vi "load_xml.vi"(8 "error in":errorcluster, 10 "child node in":refnum<k20>, 11 "Analog_Output.lvclass (in)":refnum<class "Analog_Output.lvclass">) -> (0 "error out":errorcluster, 2 "child node out":refnum<k20>, 3 "Analog_Output.lvclass":refnum<class "Analog_Output.lvclass">)   [LabVIEW 2014, in "Analog_Output.lvclass"]
doc: "Loads analog output settings from xml. Expected format:\n\n<Enable>%b</Enable>\n<PhysicalChannel>%s</PhysicalChannel>\n<MinimumValue>%f</MinimumValue>\n<MaximumValue>%f</MaximumValue>\n<SamplesPerSecond>%f</SamplesPerSecond>\n<TotalAOTime units=\"seconds\">%s</TotalAOTime>\n<AnalogOutputEquations>\n%s</AnalogOutputEquations>\n<StartTrigger.WaitForStartTrigger>%b</StartTrigger.WaitForStartTrigger\n<StartTrigger.source>%s</StartTrigger.source>\n<StartTrigger.edge>%s</StartTrigger.edge>\n\nMTL 2012 Dec 31"
uses:
  Analog_Output.lvclass
  Analog_Output.lvclass/Analog_Output.ctl
  Globals.vi
  <vilib>/xml/Close Reference(Node).vi
  <resource>/objmgr/DOMUserDefRef.rc
  <vilib>/xml/NI_XML.lvlib
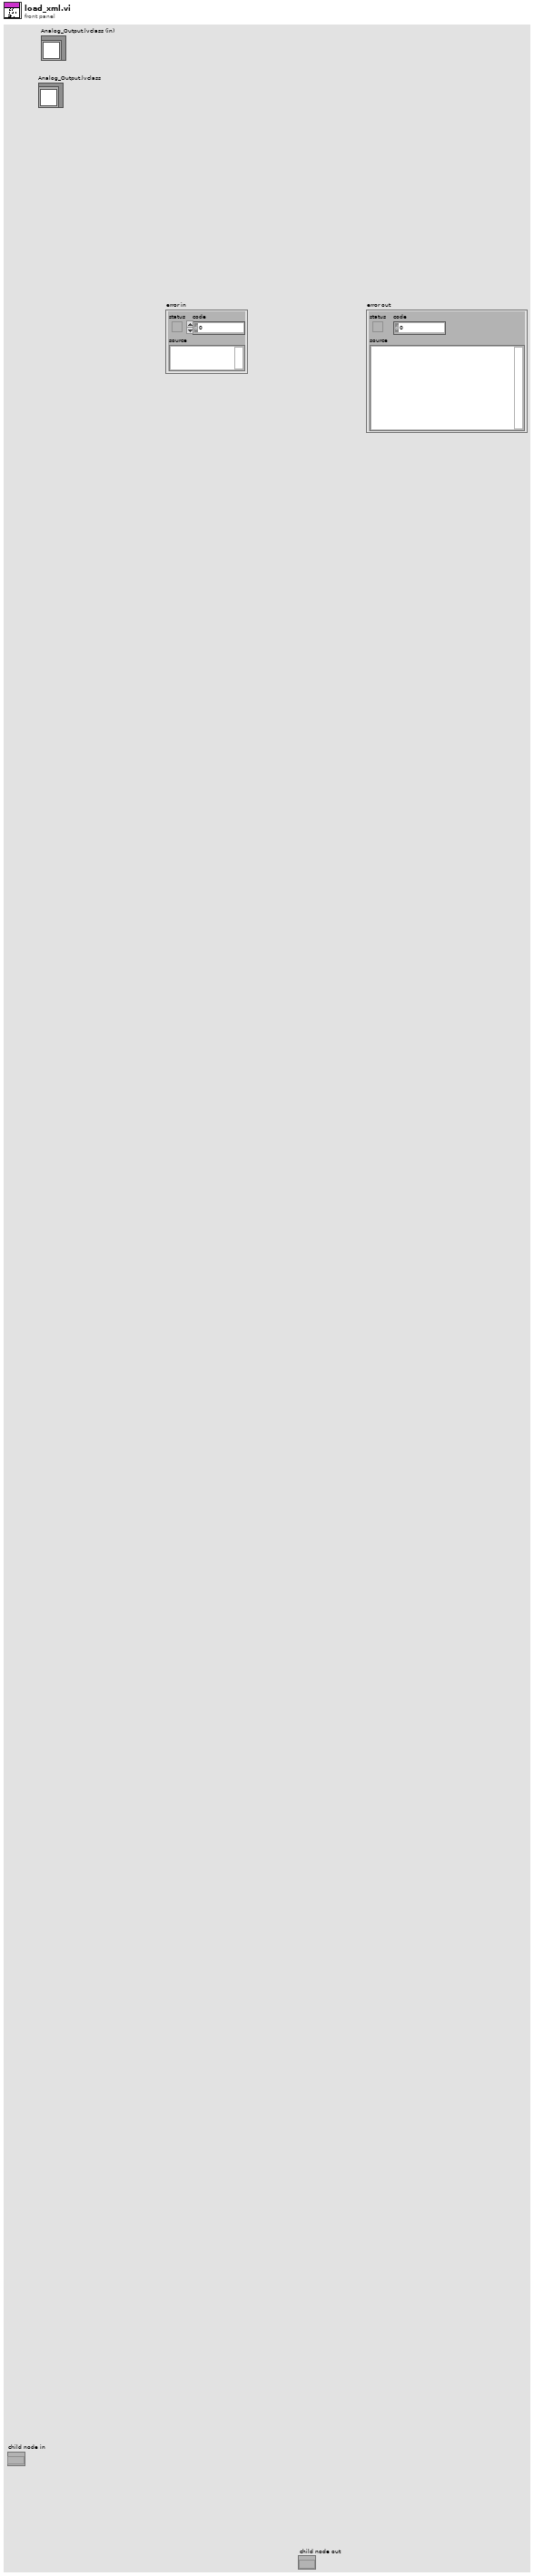
[diagram p1: front panel]
types:
  T1 = typedef "Analog_Output.lvclass/AO_settings.ctl" = cluster{"Enable Analog Out?":bool, "Physical Channel":tag, "Minimum Value":dbl, "Maximum Value":dbl, "Samples per second":dbl, "Start Trigger":cluster{"Wait for start trigger?":bool, "source":tag, "edge":i32}, "Analog Output Waveforms (channel, time)":dbl[][], "Export trigger":cluster{"Export Start Trigger?":bool, "output terminal":tag}, "External Clock":cluster{"Use external clock?":bool, "source":tag, "max expected clock rate":dbl}}
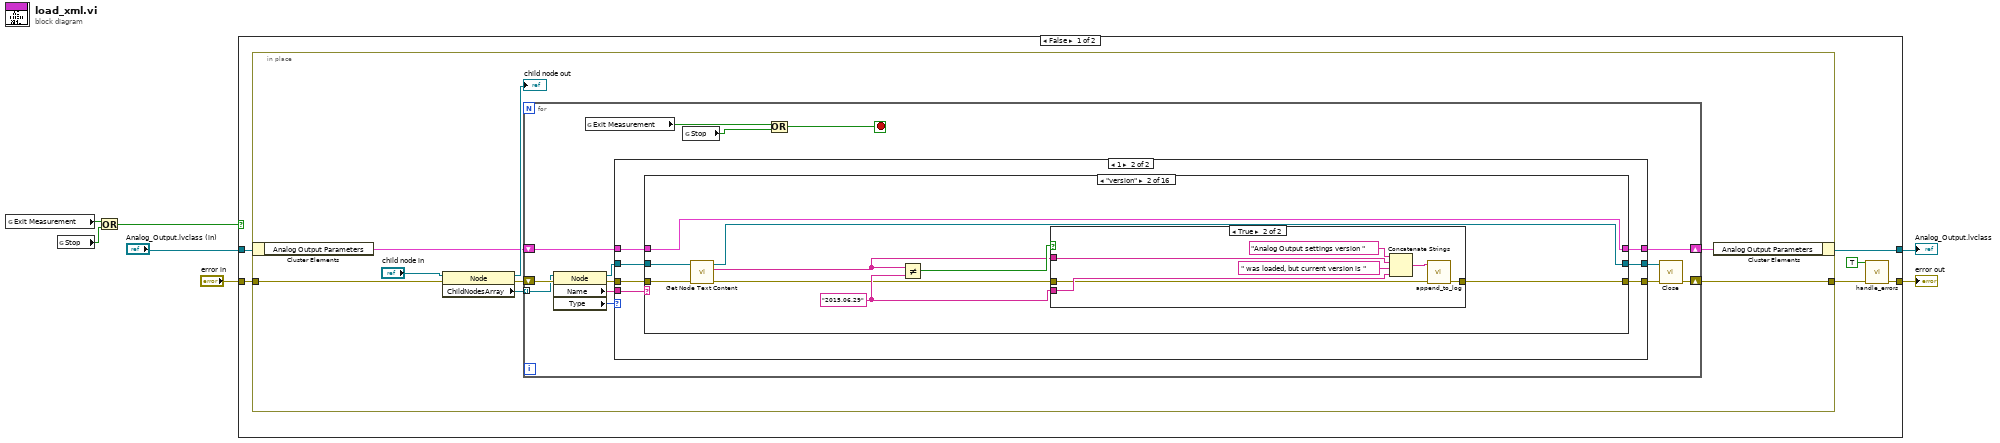
[diagram p0: block diagram]
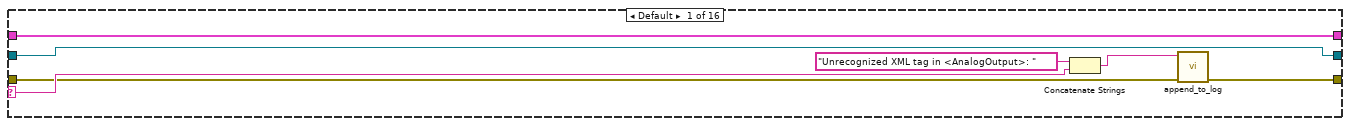
[diagram p3: hidden frame]
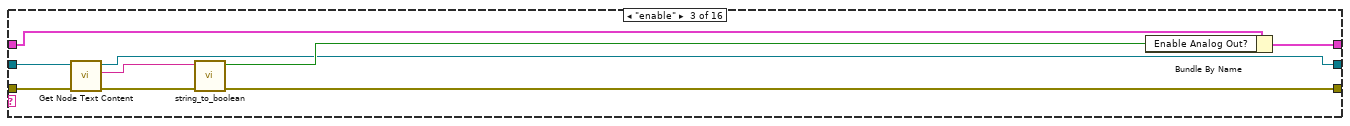
[diagram p5: hidden frame]
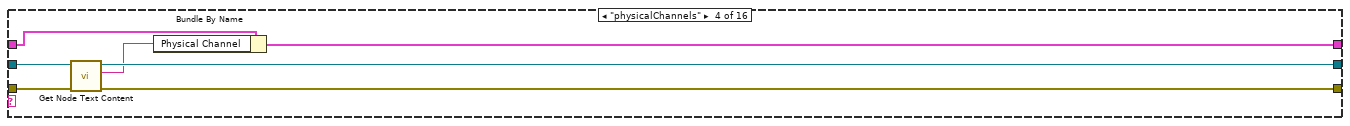
[diagram p6: hidden frame]
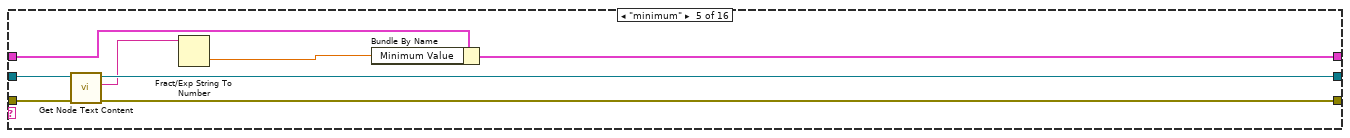
[diagram p7: hidden frame]
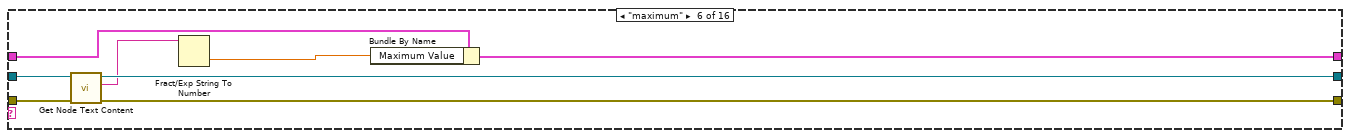
[diagram p8: hidden frame]
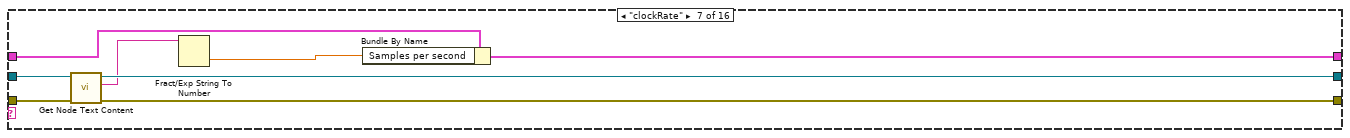
[diagram p9: hidden frame]
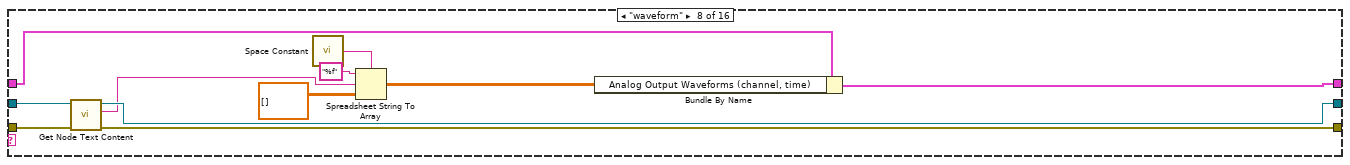
[diagram p10: hidden frame]
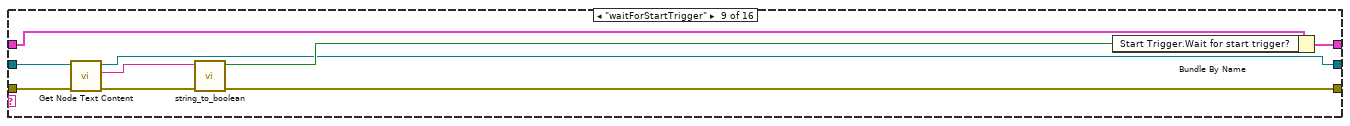
[diagram p11: hidden frame]
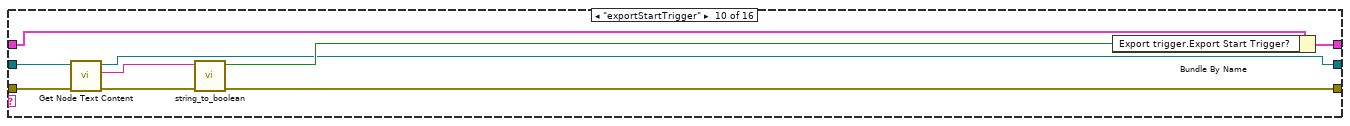
[diagram p12: hidden frame]
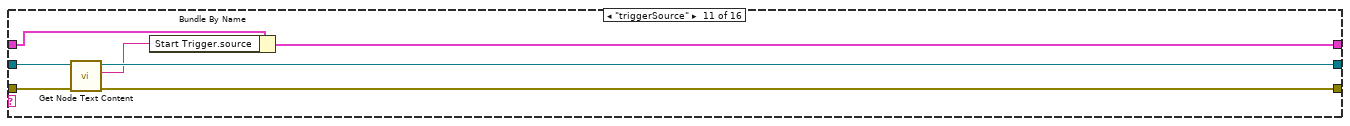
[diagram p13: hidden frame]
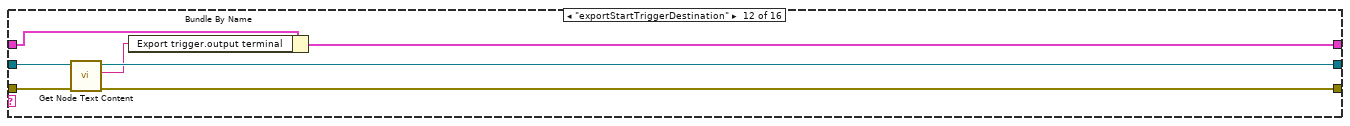
[diagram p14: hidden frame]
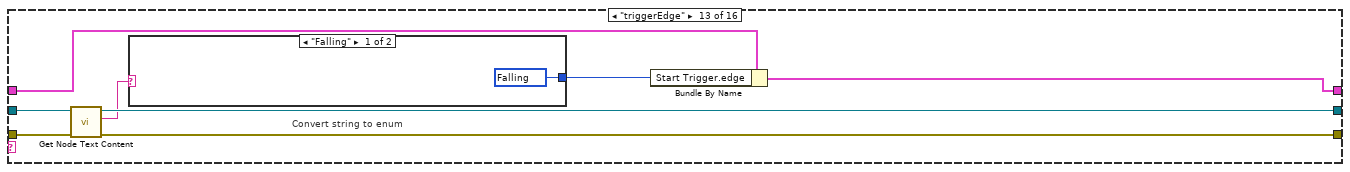
[diagram p15: hidden frame]
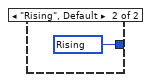
[diagram p16: hidden frame]
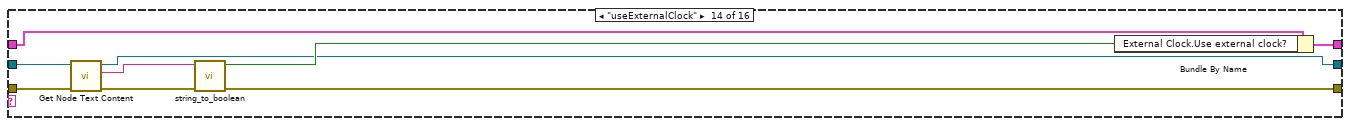
[diagram p17: hidden frame]
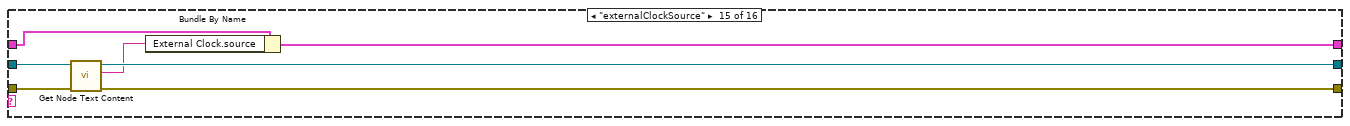
[diagram p18: hidden frame]
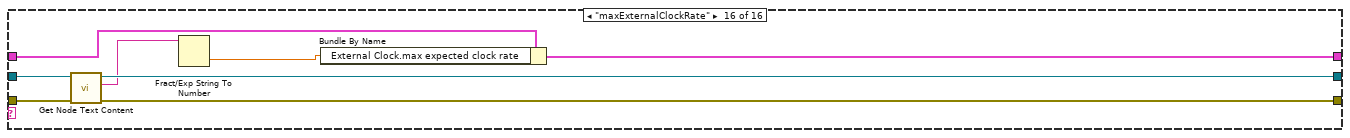
[diagram p19: hidden frame]
diagram:
  n1 = global read "Globals.vi" "Exit Measurement"() -> (w4:bool)
  n2 = global read "Globals.vi" "Stop"() -> (w3:bool)
  n3 = Or(x=w4, y=w3) -> (x .or. y?=w2:bool)
  n4 = case shown="False" w2 {
    tunnel: "Analog_Output.lvclass (in)" -> [w13 w187]
    tunnel: [w12 w187] -> w6
    tunnel: "error in" -> [w11 w188]
    tunnel: [w8 w188] -> w1
    frame False {
      n5 = in-place {
        in-place-border: w11 -> [w15]
        in-place-border: [w14] -> w10
        n6 = in-place-cluster #1(w13) -> ("Analog Output Parameters"=w16:T1)
        n7 = property class="Node"(reference="child node in", error in=w15) -> (reference out=→"child node out":refnum<k20>, error out=w19:errorcluster, "ChildNodesArray"=w21:refnum<k20>[])
        n8 = for {
          tunnel: w21 -> [w26] mode=indexing
          shift-right: [w32] -> w17
          shift-left: w16 -> [w33]
          shift-right: [w29] -> w14
          shift-left: w19 -> [w27]
          stop <- w22 stop-if-true
          n9 = property class="Node"(reference=w26, error in=w27) -> (reference out=w34:refnum<k20>, error out=w30:errorcluster, "Name"=w35:string, "Type"=w25:i32)
          n10 = global read "Globals.vi" "Exit Measurement"() -> (w24:bool)
          n11 = case shown="1" w25 {
            tunnel: w35 -> [_ w45]
            tunnel: w34 -> [w38 w44]
            tunnel: w33 -> [w36 w43]
            tunnel: [w36 w42] -> w32
            tunnel: [w38 w41] -> w31
            tunnel: w30 -> [w37 w40]
            tunnel: [w37 w39] -> w28
            frame Default {
            }
            frame 1 {
              n12 = case shown="\"version\"" w45 {
                selector: w45 -> [w48 _ _ _ _ _ _ _ _ _ _ _ _ _ _ _]
                tunnel: w44 -> [w51 w55 w78 w85 w93 w101 w109 w120 w129 w138 w145 w152 w160 w171 w178 w186]
                tunnel: w43 -> [w52 w57 w76 w83 w91 w99 w107 w118 w127 w136 w143 w150 w158 w169 w176 w184]
                tunnel: [w52 w57 w75 w82 w90 w98 w106 w117 w126 w135 w142 w149 w157 w168 w175 w183] -> w42
                tunnel: [w51 w54 w70 w81 w89 w97 w105 w116 w121 w130 w141 w148 w156 w163 w174 w182] -> w41
                tunnel: w40 -> [w47 w56 w77 w84 w92 w100 w108 w119 w128 w137 w144 w151 w159 w170 w177 w185]
                tunnel: [w46 w53 w73 w79 w88 w96 w104 w115 w124 w133 w139 w146 w155 w166 w172 w181] -> w39
                frame Default {
                  n13 = Concatenate Strings("Unrecognized XML tag in <AnalogOutput>: " ("string"), w48) -> (w49:string)
                  n14 = call "append_to_log.vi"("error in"=w47, "string"=w49) -> ("error out"=w46:errorcluster)  [unwired: 9 in]
                }
                frame "version" {
                  w59 = "2015.06.29" ("y")
                  n15 = call <vilib>:"Get Node Text Content.vi"("error in (no error)"=w56, "node in"=w55) -> ("error out"=w58:errorcluster, "node text"=w60:string, "node out"=w54:refnum<k20>)  [unwired: 7 in]
                  n16 = Not Equal?(x=w60, y=w59) -> (x != y?=w61:bool)
                  n17 = case shown="True" w61 {
                    tunnel: w60 -> [_ w68]
                    tunnel: w59 -> [_ w66]
                    tunnel: w58 -> [w62 w64]
                    tunnel: [w62 w63] -> w53
                    frame False {
                    }
                    frame True {
                      n18 = Concatenate Strings("Analog Output settings version " ("string"), w68, " was loaded, but current version is " ("string"), w66) -> (w65:string)
                      n19 = call "append_to_log.vi"("error in"=w64, "string"=w65) -> ("error out"=w63:errorcluster)  [unwired: 9 in]
                    }
                  }
                }
                frame "enable" {
                  n20 = call <vilib>:"Get Node Text Content.vi"("error in (no error)"=w77, "node in"=w78) -> ("error out"=w74:errorcluster, "node text"=w72:string, "node out"=w70:refnum<k20>)  [unwired: 7 in]
                  n21 = call "string_to_boolean.vi"("error in"=w74, "string"=w72) -> ("error out"=w73:errorcluster, "boolean"=w71:bool)  [unwired: 8 in]
                  n22 = Bundle By Name(cluster=w76, "Enable Analog Out?"=w71) -> (w75:T1)
                }
                frame "physicalChannels" {
                  n23 = call <vilib>:"Get Node Text Content.vi"("error in (no error)"=w84, "node in"=w85) -> ("error out"=w79:errorcluster, "node text"=w80:string, "node out"=w81:refnum<k20>)  [unwired: 7 in]
                  n24 = Bundle By Name(cluster=w83, "Physical Channel"=w80) -> (w82:T1)
                }
                frame "minimum" {
                  n25 = call <vilib>:"Get Node Text Content.vi"("error in (no error)"=w92, "node in"=w93) -> ("error out"=w88:errorcluster, "node text"=w87:string, "node out"=w89:refnum<k20>)  [unwired: 7 in]
                  n26 = Fract/Exp String To Number(string=w87) -> (number=w86:dbl)  [unwired: 3 in, 1 out]
                  n27 = Bundle By Name(cluster=w91, "Minimum Value"=w86) -> (w90:T1)
                }
                frame "maximum" {
                  n28 = call <vilib>:"Get Node Text Content.vi"("error in (no error)"=w100, "node in"=w101) -> ("error out"=w96:errorcluster, "node text"=w95:string, "node out"=w97:refnum<k20>)  [unwired: 7 in]
                  n29 = Fract/Exp String To Number(string=w95) -> (number=w94:dbl)  [unwired: 3 in, 1 out]
                  n30 = Bundle By Name(cluster=w99, "Maximum Value"=w94) -> (w98:T1)
                }
                frame "clockRate" {
                  n31 = call <vilib>:"Get Node Text Content.vi"("error in (no error)"=w108, "node in"=w109) -> ("error out"=w104:errorcluster, "node text"=w103:string, "node out"=w105:refnum<k20>)  [unwired: 7 in]
                  n32 = Fract/Exp String To Number(string=w103) -> (number=w102:dbl)  [unwired: 3 in, 1 out]
                  n33 = Bundle By Name(cluster=w107, "Samples per second"=w102) -> (w106:T1)
                }
                frame "waveform" {
                  n34 = call <vilib>:"Get Node Text Content.vi"("error in (no error)"=w119, "node in"=w120) -> ("error out"=w115:errorcluster, "node text"=w111:string, "node out"=w116:refnum<k20>)  [unwired: 7 in]
                  n35 = call <vilib>:"Space Constant.vi"() -> ("String"=w112:string)
                  n36 = Spreadsheet String To Array(delimiter (Tab)=w112, format string="%f", spreadsheet string=w111, array type (2D Dbl)=dbl[][] []) -> (array=w110:dbl[][])
                  n37 = Bundle By Name(cluster=w118, "Analog Output Waveforms (channel, time)"=w110) -> (w117:T1)
                }
                frame "waitForStartTrigger" {
                  n38 = call <vilib>:"Get Node Text Content.vi"("error in (no error)"=w128, "node in"=w129) -> ("error out"=w125:errorcluster, "node text"=w123:string, "node out"=w121:refnum<k20>)  [unwired: 7 in]
                  n39 = call "string_to_boolean.vi"("error in"=w125, "string"=w123) -> ("error out"=w124:errorcluster, "boolean"=w122:bool)  [unwired: 8 in]
                  n40 = Bundle By Name(cluster=w127, "Start Trigger.Wait for start trigger?"=w122) -> (w126:T1)
                }
                frame "exportStartTrigger" {
                  n41 = call <vilib>:"Get Node Text Content.vi"("error in (no error)"=w137, "node in"=w138) -> ("error out"=w134:errorcluster, "node text"=w132:string, "node out"=w130:refnum<k20>)  [unwired: 7 in]
                  n42 = call "string_to_boolean.vi"("error in"=w134, "string"=w132) -> ("error out"=w133:errorcluster, "boolean"=w131:bool)  [unwired: 8 in]
                  n43 = Bundle By Name(cluster=w136, "Export trigger.Export Start Trigger?"=w131) -> (w135:T1)
                }
                frame "triggerSource" {
                  n44 = call <vilib>:"Get Node Text Content.vi"("error in (no error)"=w144, "node in"=w145) -> ("error out"=w139:errorcluster, "node text"=w140:string, "node out"=w141:refnum<k20>)  [unwired: 7 in]
                  n45 = Bundle By Name(cluster=w143, "Start Trigger.source"=w140) -> (w142:T1)
                }
                frame "exportStartTriggerDestination" {
                  n46 = call <vilib>:"Get Node Text Content.vi"("error in (no error)"=w151, "node in"=w152) -> ("error out"=w146:errorcluster, "node text"=w147:string, "node out"=w148:refnum<k20>)  [unwired: 7 in]
                  n47 = Bundle By Name(cluster=w150, "Export trigger.output terminal"=w147) -> (w149:T1)
                }
                frame "triggerEdge" {
                  n48 = call <vilib>:"Get Node Text Content.vi"("error in (no error)"=w159, "node in"=w160) -> ("error out"=w155:errorcluster, "node text"=w154:string, "node out"=w156:refnum<k20>)  [unwired: 7 in]
                  n49 = case "Convert string to enum" shown="\"Falling\"" w154 {
                    tunnel: [w161 w162] -> w153
                    frame "Falling" {
                      w161 = 10171 items=["Rising"=10280, "Falling"=10171] ("edge")
                    }
                    frame "Rising", Default {
                      w162 = 10280 items=["Rising"=10280, "Falling"=10171] ("edge")
                    }
                  }
                  n50 = Bundle By Name(cluster=w158, "Start Trigger.edge"=w153) -> (w157:T1)
                }
                frame "useExternalClock" {
                  n51 = call <vilib>:"Get Node Text Content.vi"("error in (no error)"=w170, "node in"=w171) -> ("error out"=w167:errorcluster, "node text"=w165:string, "node out"=w163:refnum<k20>)  [unwired: 7 in]
                  n52 = call "string_to_boolean.vi"("error in"=w167, "string"=w165) -> ("error out"=w166:errorcluster, "boolean"=w164:bool)  [unwired: 8 in]
                  n53 = Bundle By Name(cluster=w169, "External Clock.Use external clock?"=w164) -> (w168:T1)
                }
                frame "externalClockSource" {
                  n54 = call <vilib>:"Get Node Text Content.vi"("error in (no error)"=w177, "node in"=w178) -> ("error out"=w172:errorcluster, "node text"=w173:string, "node out"=w174:refnum<k20>)  [unwired: 7 in]
                  n55 = Bundle By Name(cluster=w176, "External Clock.source"=w173) -> (w175:T1)
                }
                frame "maxExternalClockRate" {
                  n56 = call <vilib>:"Get Node Text Content.vi"("error in (no error)"=w185, "node in"=w186) -> ("error out"=w181:errorcluster, "node text"=w180:string, "node out"=w182:refnum<k20>)  [unwired: 7 in]
                  n57 = Fract/Exp String To Number(string=w180) -> (number=w179:dbl)  [unwired: 3 in, 1 out]
                  n58 = Bundle By Name(cluster=w184, "External Clock.max expected clock rate"=w179) -> (w183:T1)
                }
              }
            }
          }
          n59 = global read "Globals.vi" "Stop"() -> (w23:bool)
          n60 = Or(x=w24, y=w23) -> (x .or. y?=w22:bool)
          n61 = call-poly <vilib>:"Close.vi"("error in (no error)"=w28, "node"=w31) -> ("error out"=w29:errorcluster)  [unwired: 7 in]
        }
        n62 = in-place-cluster #1("Analog Output Parameters"=w17) -> (w12:refnum<class "Analog_Output.lvclass">)
      }
      n63 = call "handle_errors.vi"("Exit Operation"=TRUE, "error in (no error)"=w10) -> ("error out"=w8:errorcluster)  [unwired: 13 in]
    }
    frame True {
    }
  }
  "Analog_Output.lvclass" <- w6
  "error out" <- w1
